vi "InitPort.vi"(8 "error in (no error)":errorcluster, 9 "Скорость передачи":u32, 10 "Порт":refnum<visa-resource-name>) -> (0 "error out":errorcluster, 3 "StepMotor out":refnum<class "StepMotor.lvclass">)   [LabVIEW 2010, in "StepMotor.lvclass"]
uses:
  StepMotor.lvclass
  StepMotor.lvclass/StepMotor.ctl
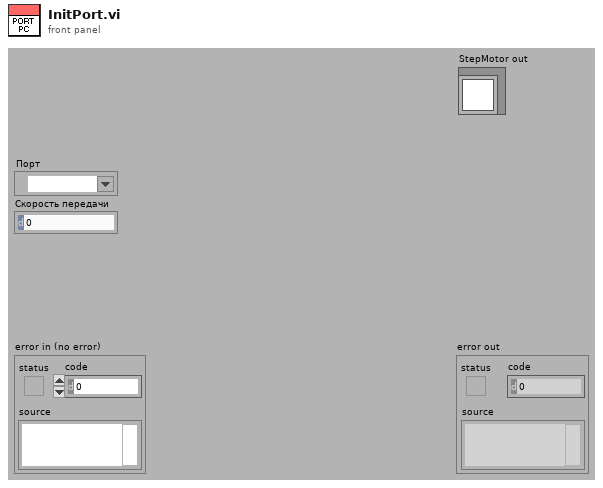
[diagram p1: front panel]
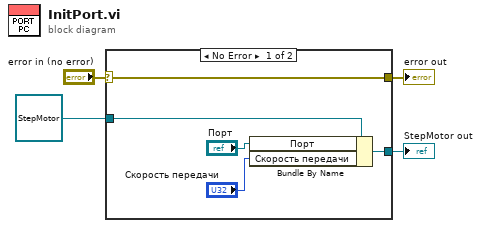
[diagram p0: block diagram]
diagram:
  n1 = case shown="No Error" "error in (no error)" {
    selector: "error in (no error)" -> [w5 w11]
    tunnel: [w5 w11] -> w3
    tunnel: refnum<class "StepMotor.lvclass"> refnum ("StepMotor.lvclass") -> [w7 w10]
    tunnel: [w6 w10] -> w2
    frame No Error {
      n2 = Bundle By Name(cluster=w7, "Порт"="Порт", "Скорость передачи"="Скорость передачи") -> (w6:refnum<class "StepMotor.lvclass">)
    }
    frame Error {
    }
  }
  "StepMotor out" <- w2
  "error out" <- w3
